vi "FITS_ReadU16.vi"(8 "error in (no error)":errorcluster, 9 "Plane# (0..n-1)":u16, 10 "FITS":T2={"BITPIX"=8, "NAXIS"=2, "NAXIS1"=1, "NAXIS2"=1, "NAXIS3"=1, "BZERO"=0.0, "BSCALE"=1.0}, 11 "FITS file":T1) -> (0 "error out":errorcluster, 2 "Array":u16[][](array[numeric]), 3 "Byte Stream File out":refnum<file>)   [LabVIEW 2011]
panel:
  out "Pixels":dbl
  # "0/0 ist wohl links unten?!"
  # "x"
  # "y"
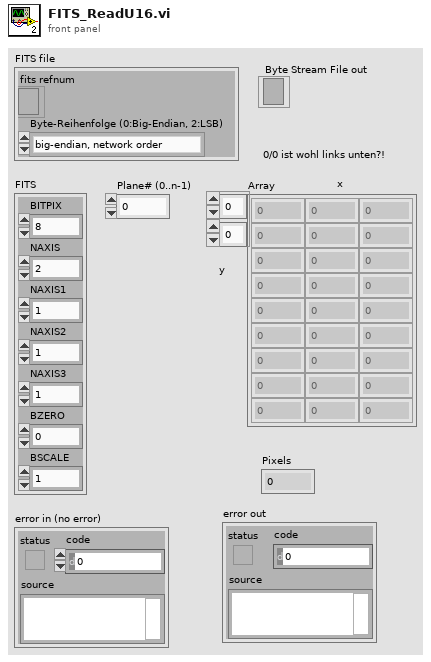
[diagram p1: front panel]
types:
  T1 = cluster{"fits refnum":refnum<file>, "Byte-Reihenfolge (0:Big-Endian, 2:LSB)":enum16{"big-endian, network order", "native, host order", "little-endian"}}
  T2 = cluster{"BITPIX":i16, "NAXIS":i16, "NAXIS1":u16, "NAXIS2":u16, "NAXIS3":u16, "BZERO":dbl, "BSCALE":dbl}
  T3 = enum16{"big-endian, network order", "native, host order", "little-endian"}
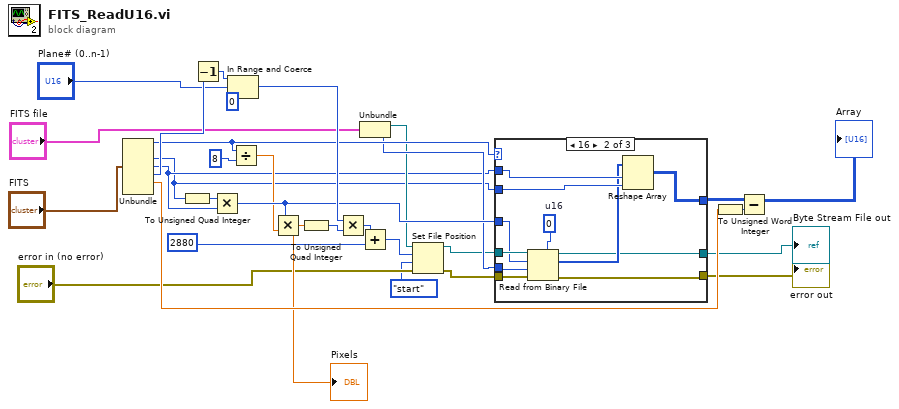
[diagram p0: block diagram]
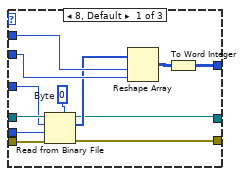
[diagram p2: hidden frame]
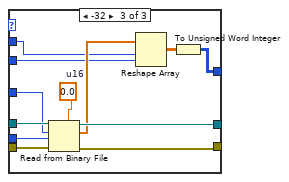
[diagram p3: hidden frame]
diagram:
  n1 = Unbundle("FITS") -> ("BITPIX"=w21:i16, "NAXIS1"=w1:u16, "NAXIS2"=w2:u16, "NAXIS3"=w25:u16, "BZERO"=w29:dbl)  [unwired: 2 out]
  n2 = To Unsigned Quad Integer(1:w1) -> (0:w22:u64)
  n3 = Decrement(x=w25) -> (x-1=w26:u16)
  n4 = Multiply(x=w22, y=w2) -> (x*y=w16:u64)
  n5 = In Range and Coerce(upper limit=w26, x="Plane# (0..n-1)", lower limit=u16 0) -> (coerced(x)=w23:u16)  [unwired: 1 out]
  n6 = Divide(x=w21, y=i16 8) -> (x/y=w15:dbl)
  n7 = Multiply(x=w16, y=w15) -> (x*y=w17:dbl)
  "Pixels" <- w17
  n8 = To Unsigned Quad Integer(1:w17) -> (0:w19:u64)
  n9 = Multiply(x=w23, y=w19) -> (x*y=w18:u64)
  n10 = Unbundle("FITS file") -> ("fits refnum"=w7:refnum<file>, "Byte-Reihenfolge (0:Big-Endian, 2:LSB)"=w11:T3)
  n11 = Add(x=w18, y=2880) -> (x+y=w8:u64)
  n12 = Set File Position(offset (in bytes) (0)=w8, refnum=w7, from (0:start)=enum16{"start", "end", "current"}."start" ("pos mode (0:2)"), error in="error in (no error)") -> (refnum out=w10:refnum<file>, error out=w5:errorcluster)
  n13 = case shown="16" w21 {
    tunnel: w2 -> [w43 w54 w58]
    tunnel: w1 -> [w42 w53 w57]
    tunnel: [w33 w52 w55] -> w28
    tunnel: w10 -> [w40 w51 w65]
    tunnel: w5 -> [w39 w50 w64]
    tunnel: [w38 w47 w61] -> w12
    tunnel: w16 -> [w35 w45 w62]
    tunnel: w11 -> [w34 w49 w63]
    tunnel: [w32 w44 w60] -> w13
    frame 8, Default {
      w36 = u8 0  # Byte
      n14 = Read from Binary File(5:w36, 8:w39, 9:w34, 10:w35, 11:w40) -> (0:w38:errorcluster, 2:w37:u8[], 3:w32:refnum<file>)  [unwired: 2 out]
      n15 = Reshape Array(w37, w43, w42) -> (w41:u8[][])
      n16 = To Word Integer(number=w41) -> (16bit integer=w33:i16[][])
    }
    frame 16 {
      w48 = u16 0  # u16
      n17 = Read from Binary File(5:w48, 8:w50, 9:w49, 10:w45, 11:w51) -> (0:w47:errorcluster, 2:w46:u16[], 3:w44:refnum<file>)  [unwired: 2 out]
      n18 = Reshape Array(w46, w54, w53) -> (w52:u16[][])
    }
    frame -32 {
      w66 = sgl 0.0  # u16
      n19 = Read from Binary File(5:w66, 8:w64, 9:w63, 10:w62, 11:w65) -> (0:w61:errorcluster, 2:w59:sgl[], 3:w60:refnum<file>)  [unwired: 2 out]
      n20 = Reshape Array(w59, w58, w57) -> (w56:sgl[][])
      n21 = To Unsigned Word Integer(number=w56) -> (unsigned 16bit integer=w55:u16[][])
    }
  }
  "Byte Stream File out" <- w13
  "error out" <- w12
  n22 = To Unsigned Word Integer(number=w29) -> (unsigned 16bit integer=w30:u16)
  n23 = Subtract(x=w28, y=w30) -> (x-y=→"Array":u16[][])
